vi "Update Direction Parameters.vi"(8 "error in (no error)":errorcluster, 11 "senseHatDisplay in":refnum<class "RPI.SenseHat.Display.lvclass">) -> (0 "error out":errorcluster, 3 "senseHatDisplay out":refnum<class "RPI.SenseHat.Display.lvclass">)   [LabVIEW 2020, in "RPI.SenseHat.Display.lvlib" / "RPI.SenseHat.Display.lvclass"]
uses:
  RPI.SenseHat.Display.lvclass
  RPI.SenseHat.Display.lvclass/RPI.SenseHat.Display.ctl
  RPI.SenseHat.Display.lvlib
  Image/Image.lvclass
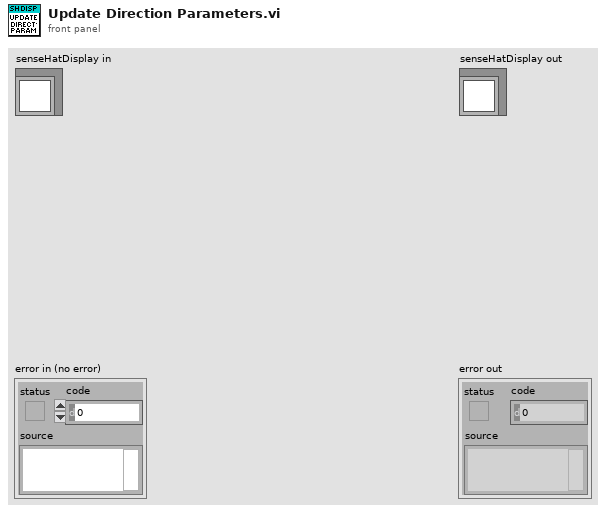
[diagram p1: front panel]
types:
  T1 = typedef "RPI.SenseHat.Display.lvlib/direction.ctl" = enum16{"deg0", "deg90", "deg180", "deg270"}
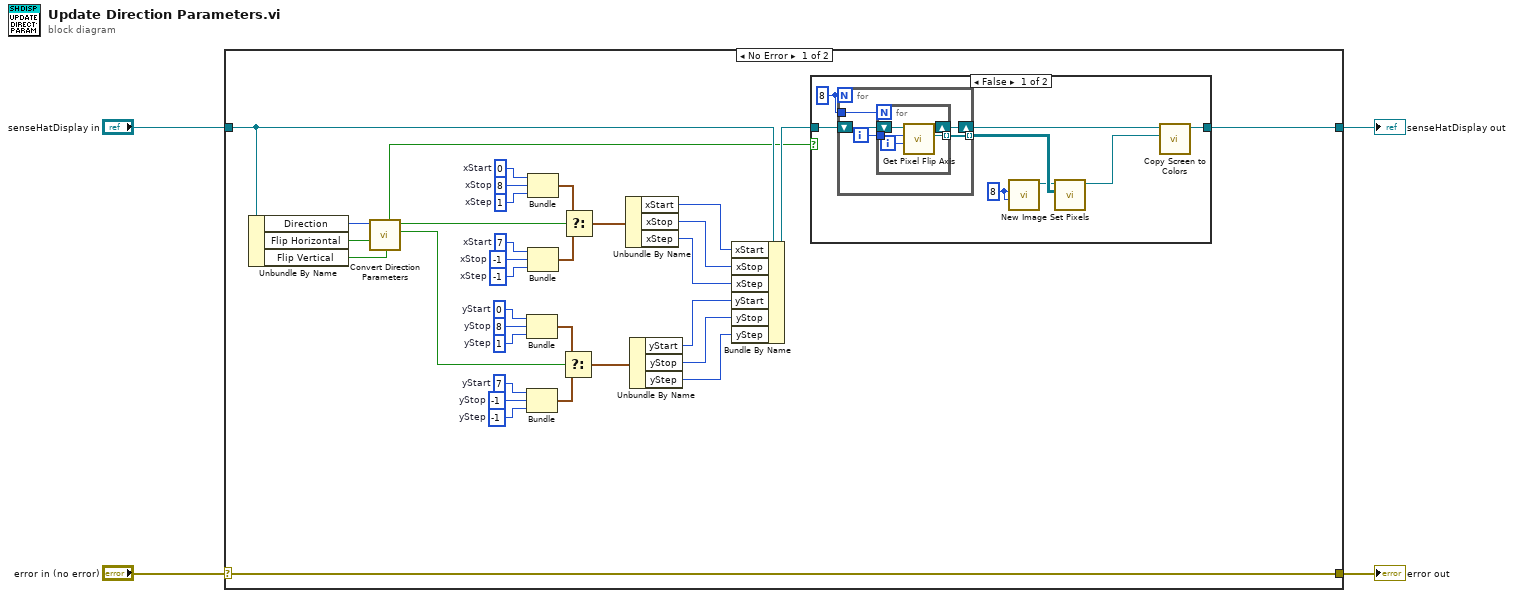
[diagram p0: block diagram]
diagram:
  n1 = case shown="No Error" "error in (no error)" {
    selector: "error in (no error)" -> [w38 w59]
    tunnel: [w38 w59] -> w3
    tunnel: [w6 w58] -> w1
    tunnel: "senseHatDisplay in" -> [w34 w58]
    frame No Error {
      w21 = -1  # yStep
      w22 = -1  # yStop
      w23 = 7  # yStart
      w19 = 1  # yStep
      w18 = 8  # yStop
      w17 = 0  # yStart
      w28 = -1  # xStep
      w27 = -1  # xStop
      w26 = 7  # xStart
      w30 = 1  # xStep
      w31 = 8  # xStop
      w32 = 0  # xStart
      n2 = Unbundle By Name(w34) -> ("Direction"=w37:T1, "Flip Horizontal"=w36:bool, "Flip Vertical"=w35:bool)
      n3 = call "Convert Direction Parameters.vi"("Flip Vertical"=w35, "Flip Horizontal"=w36, "Display Direction"=w37) -> ("Top To Bottom"=w16:bool, "Left To Right"=w33:bool, "Flip Axis"=w5:bool)  [unwired: 6 in]
      n4 = Bundle("yStart"=w17, "yStop"=w18, "yStep"=w19) -> (w20:cluster{"yStart":i32, "yStop":i32, "yStep":i32})  [unwired: 1 in]
      n5 = Bundle("yStart"=w23, "yStop"=w22, "yStep"=w21) -> (w24:cluster{"yStart":i32, "yStop":i32, "yStep":i32})  [unwired: 1 in]
      n6 = Bundle("xStart"=w32, "xStop"=w31, "xStep"=w30) -> (w29:cluster{"xStart":i32, "xStop":i32, "xStep":i32})  [unwired: 1 in]
      n7 = Bundle("xStart"=w26, "xStop"=w27, "xStep"=w28) -> (w25:cluster{"xStart":i32, "xStop":i32, "xStep":i32})  [unwired: 1 in]
      n8 = Select(t=w20, s=w16, f=w24) -> (s? t:f=w11:cluster{"yStart":i32, "yStop":i32, "yStep":i32})
      n9 = Select(t=w29, s=w33, f=w25) -> (s? t:f=w15:cluster{"xStart":i32, "xStop":i32, "xStep":i32})
      n10 = Unbundle By Name(w15) -> ("xStart"=w14:i32, "xStop"=w13:i32, "xStep"=w12:i32)
      n11 = Unbundle By Name(w11) -> ("yStart"=w10:i32, "yStop"=w9:i32, "yStep"=w8:i32)
      n12 = Bundle By Name(cluster=w34, "xStart"=w14, "xStop"=w13, "xStep"=w12, "yStart"=w10, "yStop"=w9, "yStep"=w8) -> (w7:refnum<class "RPI.SenseHat.Display.lvclass">)
      n13 = case shown="False" w5 {
        tunnel: w7 -> [w46 w57]
        tunnel: [w44 w57] -> w6
        frame False {
          w39 = 8
          w40 = 8 ("Width")
          n14 = for {
            N: w39 -> [_]
            shift-right: [w50] -> w45
            shift-left: w46 -> [w49]
            tunnel: [w48] -> w43 mode=indexing
            tunnel: w39 -> [w47]
            i -> [w51]
            n15 = for {
              N: w47 -> [_]
              tunnel: w51 -> [w55]
              shift-right: [w54] -> w50
              shift-left: w49 -> [w53]
              tunnel: [w52] -> w48 mode=indexing
              i -> [w56]
              n16 = call "Get Pixel Flip Axis.vi"("y"=w56, "x"=w55, "senseHatDisplay in"=w53) -> ("Pixel"=w52:refnum<class "Pixel.lvclass">, "senseHatDisplay out"=w54:refnum<class "RPI.SenseHat.Display.lvclass">)  [unwired: 6 in, 1 out]
            }
          }
          n17 = call "New Image.vi"("Height"=w40, "Width"=w40) -> ("Image out"=w41:refnum<class "Image.lvclass">)  [unwired: 8 in, 1 out]
          n18 = call "Set Pixels.vi"("Pixels"=w43, "Image in"=w41) -> ("Image out"=w42:refnum<class "Image.lvclass">)  [unwired: 8 in, 1 out]
          n19 = call "Copy Screen to Colors.vi"("Image"=w42, "senseHatDisplay in"=w45) -> ("senseHatDisplay out"=w44:refnum<class "RPI.SenseHat.Display.lvclass">)  [unwired: 8 in, 1 out]
        }
        frame True {
        }
      }
    }
    frame Error {
    }
  }
  "error out" <- w3
  "senseHatDisplay out" <- w1
